vi "PAQ_Table_read_samples_Selection.vi"(5 "Time-End":timestamp, 7 "Time-Start":timestamp, 8 "error in (no error)":errorcluster, 9 "Sub Path":path, 11 "Table Filename":string) -> (0 "error out":errorcluster, 1 "TAGs":string[](array[string]), 2 "Fetched samples":i32, 3 "Fetched PAQ-samples":T1)   [LabVIEW 2020, in "Sgraph_lib_V1.lvlib" / "DBAL-BIN.lvclass"]
doc: "Read all samples from one PAQ file"
uses:
  DBAL-BIN.lvclass
  controls/BIN/BINdata.ctl
panel:
  out "time Arr":timestamp[](array[timestamp])
  out "MinGet":timestamp
  out "MaxGet":timestamp
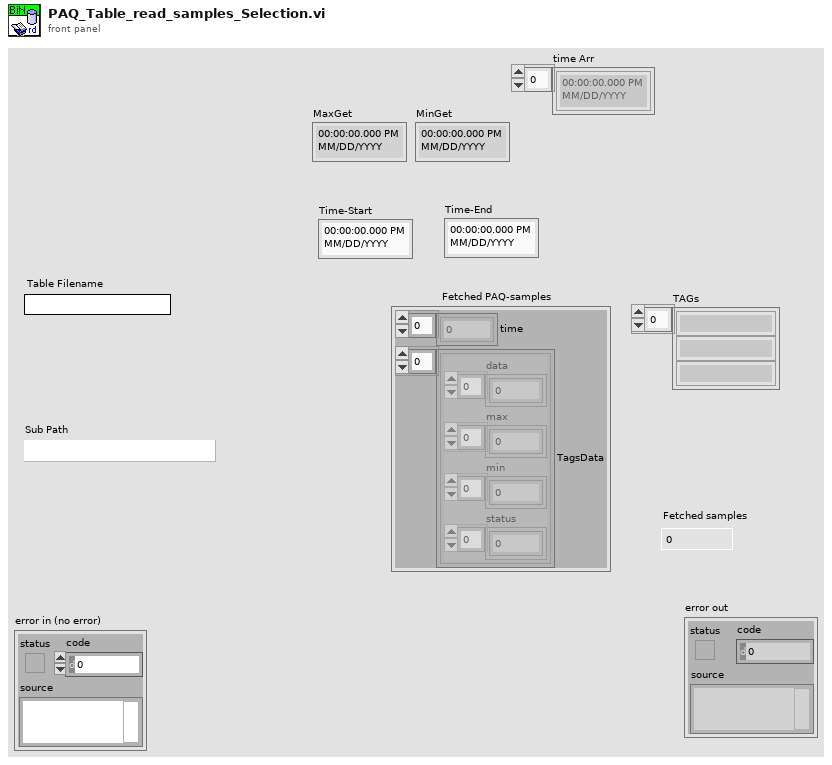
[diagram p1: front panel]
types:
  T1 = typedef "Sgraph_lib_V1.lvlib/DBAL-BIN.lvclass/BINdata.ctl" = cluster{"time":dbl[], "TagsData":cluster{"data":dbl[], "max":dbl[], "min":dbl[], "status":u32[]}[]}
  T2 = cluster{"data":dbl[], "max":dbl[], "min":dbl[], "status":u32[]}[]
  T3 = cluster{"data":dbl[], "max":dbl[], "min":dbl[], "status":u32[]}
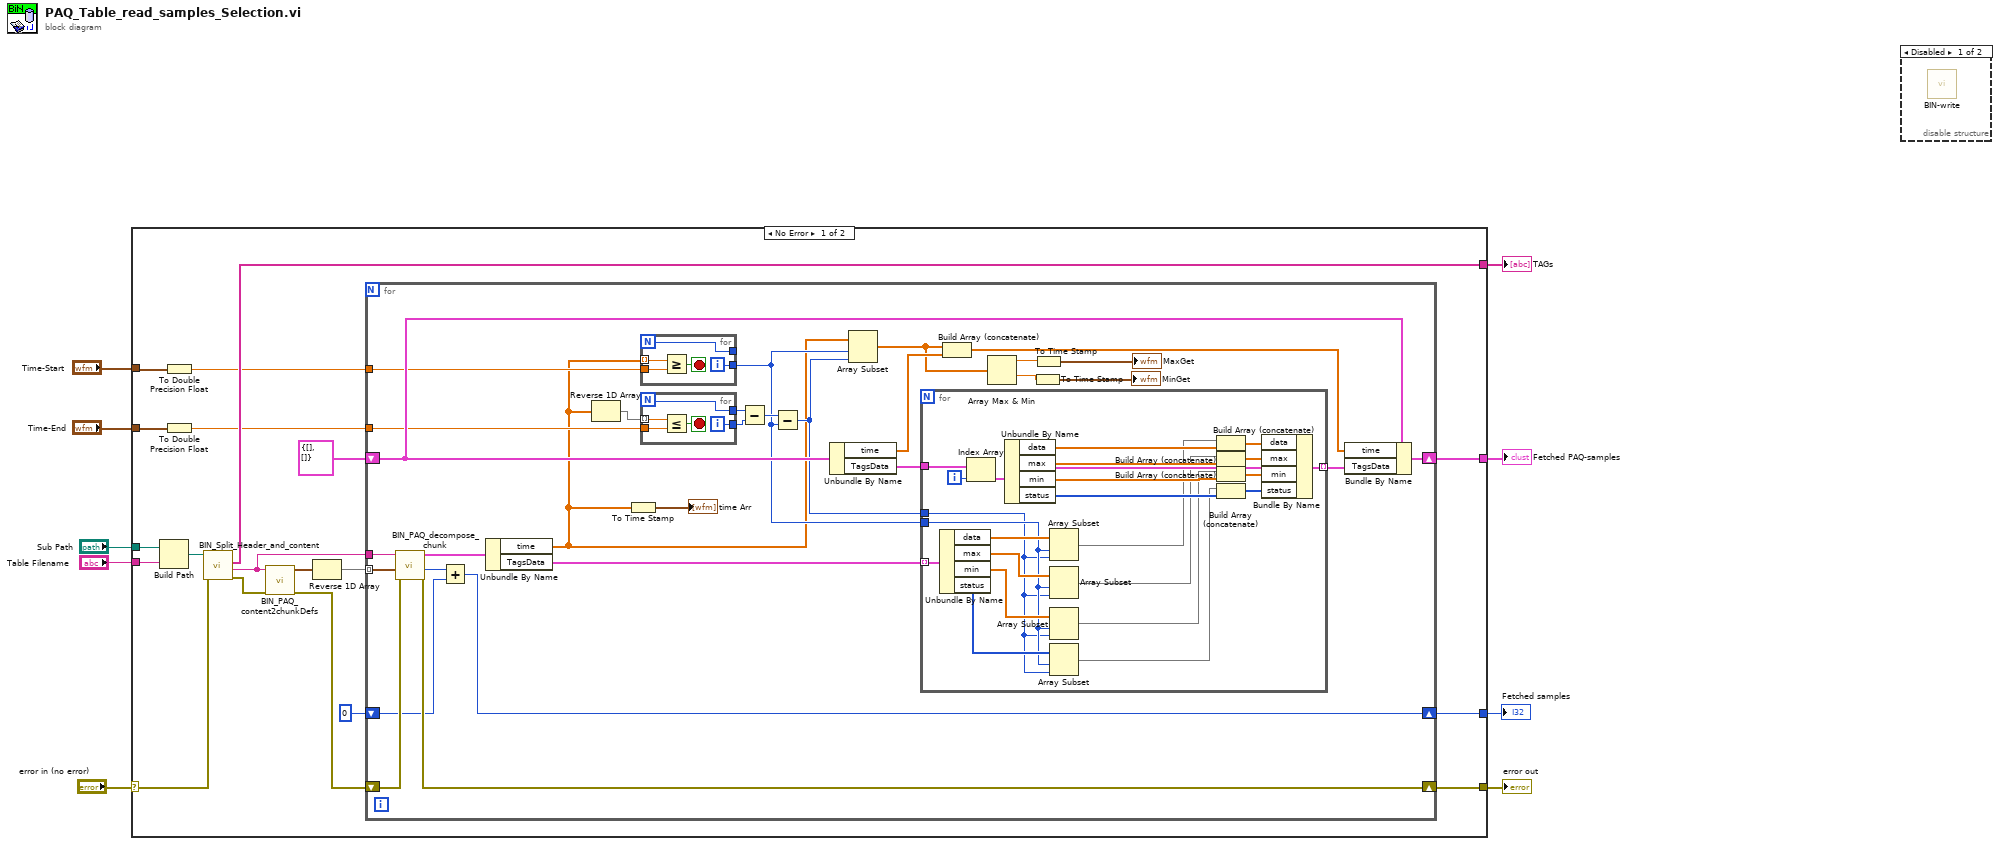
[diagram p0: block diagram]
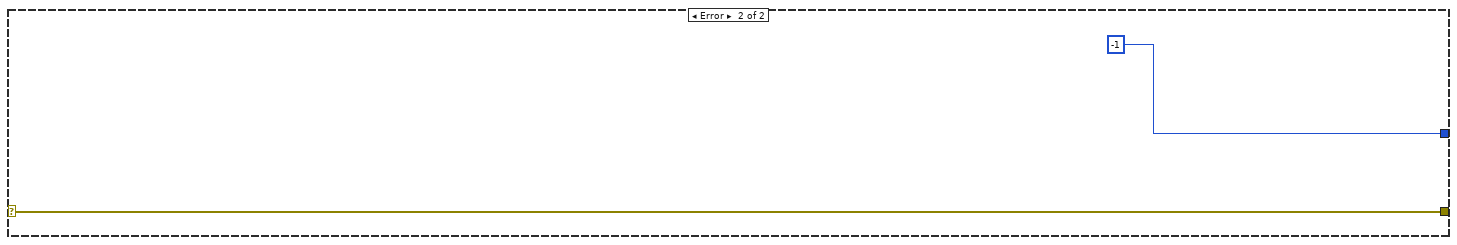
[diagram p3: hidden frame]
diagram:
  n1 = case shown="No Error" "error in (no error)" {
    selector: "error in (no error)" -> [w27 w93]
    tunnel: [w23 w93] -> w8
    tunnel: "Sub Path" -> [w15 _]
    tunnel: "Table Filename" -> [w14 _]
    tunnel: [w18 -1 ("Samples size")] -> w3
    tunnel: [w17 _] -> w5
    tunnel: [w16 _] -> w4
    tunnel: "Time-Start" -> [w13 _]
    tunnel: "Time-End" -> [w12 _]
    frame No Error {
      n2 = Build Path(base path=w15, name or relative path=w14) -> (appended path=w28:path)
      n3 = To Double Precision Float(number=w13) -> (double precision float=w10:dbl)
      n4 = To Double Precision Float(number=w12) -> (double precision float=w11:dbl)
      n5 = call "BIN_Split_Header_and_content.vi"("error in"=w27, "Path in"=w28) -> ("error out"=w26:errorcluster, "Content"=w25:string, "TAGs"=w16:string[])  [unwired: 5 in, 2 out]
      n6 = call "BIN_PAQ_content2chunkDefs.vi"("error in (no error)"=w26, "Content"=w25) -> ("error out"=w24:errorcluster, "Data segments"=w22:cluster{"Offset":u32, "Size":u32}[])  [unwired: 8 in]
      n7 = Reverse 1D Array(array=w22) -> (reversed array=w21:cluster{"Offset":u32, "Size":u32}[])
      n8 = for {
        tunnel: w21 -> [w58] mode=indexing
        tunnel: w25 -> [w57]
        shift-right: [w55] -> w23
        shift-left: w24 -> [w56]
        shift-right: [w46] -> w18
        shift-left: 0 ("Samples size") -> [w48]
        shift-right: [w53] -> w17
        shift-left: T1 {"time"=[], "TagsData"=[]} ("PAQ_data") -> [w54]
        tunnel: w11 -> [w45]
        tunnel: w10 -> [w42]
        n9 = call "BIN_PAQ_decompose_chunk.vi"("error in (no error)"=w56, "Offset"=w58, "Content"=w57) -> ("error out"=w55:errorcluster, "Samples size"=w49:i32, "PAQ_data"=w40:T1)  [unwired: 6 in]
        n10 = Add(x=w49, y=w48) -> (x+y=w46:i32)
        n11 = Unbundle By Name(w40) -> ("time"=w30:dbl[], "TagsData"=w34:T2)
        n12 = Reverse 1D Array(array=w30) -> (reversed array=w29:dbl[])
        n13 = To Time Stamp(1:w30) -> (0:→"time Arr":timestamp[])
        n14 = for {
          N -> [w60]
          tunnel: w30 -> [w63] mode=indexing
          tunnel: w42 -> [w62]
          tunnel: [w60] -> _
          tunnel: [w59] -> w33
          i -> [w59]
          stop <- w61 stop-if-true
          n15 = Greater Or Equal?(x=w63, y=w62) -> (x >= y?=w61:bool)
        }
        n16 = for {
          N -> [w65]
          tunnel: w29 -> [w68] mode=indexing
          tunnel: w45 -> [w67]
          tunnel: [w65] -> w44
          tunnel: [w64] -> w43
          i -> [w64]
          stop <- w66 stop-if-true
          n17 = Less Or Equal?(x=w68, y=w67) -> (x <= y?=w66:bool)
        }
        n18 = Subtract(x=w44, y=w43) -> (x-y=w41:i32)
        n19 = Subtract(x=w41, y=w33) -> (x-y=w32:i32)
        n20 = Unbundle By Name(w54) -> ("time"=w52:dbl[], "TagsData"=w51:T2)
        n21 = Array Subset(array=w30, index=w33, length=w32) -> (w39:dbl[])
        n22 = for {
          tunnel: w34 -> [w89] mode=indexing
          tunnel: w51 -> [w91]
          tunnel: [w83] -> w50 mode=indexing
          tunnel: w33 -> [w74]
          tunnel: w32 -> [w73]
          i -> [w90]
          n23 = Unbundle By Name(w89) -> ("data"=w78:dbl[], "max"=w77:dbl[], "min"=w76:dbl[], "status"=w75:u32[])
          n24 = Index Array(array=w91, index=w90) -> (element=w84:T3)
          n25 = Unbundle By Name(w84) -> ("data"=w88:dbl[], "max"=w87:dbl[], "min"=w86:dbl[], "status"=w85:u32[])
          n26 = Array Subset(array=w78, index=w74, length=w73) -> (w72:dbl[])
          n27 = Array Subset(array=w77, index=w74, length=w73) -> (w71:dbl[])
          n28 = Array Subset(array=w76, index=w74, length=w73) -> (w70:dbl[])
          n29 = Array Subset(array=w75, index=w74, length=w73) -> (w69:u32[])
          n30 = Build Array (concatenate)(w72, w88) -> (w80:dbl[])
          n31 = Build Array (concatenate)(w71, w87) -> (w81:dbl[])
          n32 = Build Array (concatenate)(w70, w86) -> (w82:dbl[])
          n33 = Build Array (concatenate)(w69, w85) -> (w79:u32[])
          n34 = Bundle By Name(cluster=w84, "data"=w80, "max"=w81, "min"=w82, "status"=w79) -> (w83:T3)
        }
        n35 = Build Array (concatenate)(w39, w52) -> (w47:dbl[])
        n36 = Array Max & Min(array=w39) -> (max value=w38:dbl, min value=w37:dbl)  [unwired: 2 out]
        n37 = To Time Stamp(1:w37) -> (0:→"MinGet":timestamp)
        n38 = To Time Stamp(1:w38) -> (0:→"MaxGet":timestamp)
        n39 = Bundle By Name(cluster=w54, "time"=w47, "TagsData"=w50) -> (w53:T1)
      }
    }
    frame Error {
    }
  }
  "error out" <- w8
  "Fetched samples" <- w3
  "TAGs" <- w4
  "Fetched PAQ-samples" <- w5
  n40 = disable-structure shown="Disabled" {
    frame Disabled {
      n41 = call "BIN-write.vi"() -> ()  [unwired: 9 in, 3 out]
    }
    frame Enabled {
    }
  }
